vi "Get ni_measurements_v1_MeasurementParameters.vi"(8 "error in (no error)":errorcluster, 11 "gRPCid":T5) -> (0 "error out":errorcluster, 2 "package_templatemessage":T1, 3 "gRPCid out":T5)   [LabVIEW 2020, in "LoadRegulation.lvlib"]
uses:
  LoadRegulation.lvlib
  a51dd2a7-b5c1-4c09-9df4-8cd9d3bd0c19.vi
  ni_measurements_v1_ConfigurationParameter.ctl
  google_protobuf_Any.ctl
  ni_measurements_v1_Output.ctl
  ni_measurements_v1_MeasurementParameters.ctl
  <vilib>/gRPC/LabVIEW gRPC Library/Server API/typeDefs/grpcId.ctl
  <vilib>/gRPC/LabVIEW gRPC Library/gprc-lvsupport-release.lvlib
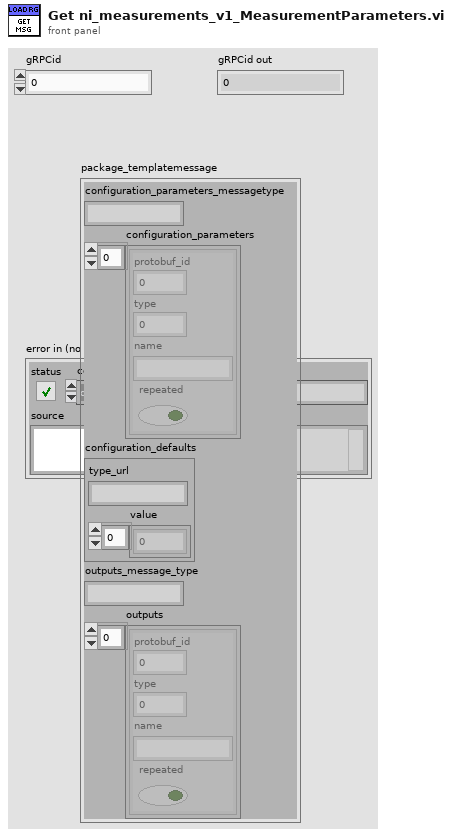
[diagram p1: front panel]
types:
  T1 = typedef "LoadRegulation.lvlib/ni_measurements_v1_MeasurementParameters.ctl" = cluster{"configuration_parameters_messagetype":string, "configuration_parameters":T2[], "configuration_defaults":T3, "outputs_message_type":string, "outputs":T4[]}
  T2 = typedef "LoadRegulation.lvlib/ni_measurements_v1_ConfigurationParameter.ctl" = cluster{"protobuf_id":u32, "type":i32, "name":string, "repeated":bool}
  T3 = typedef "LoadRegulation.lvlib/google_protobuf_Any.ctl" = cluster{"type_url":string, "value":u8[]}
  T4 = typedef "LoadRegulation.lvlib/ni_measurements_v1_Output.ctl" = cluster{"protobuf_id":u32, "type":i32, "name":string, "repeated":bool}
  T5 = typedef "gprc-lvsupport-release.lvlib/grpcId.ctl" = u64
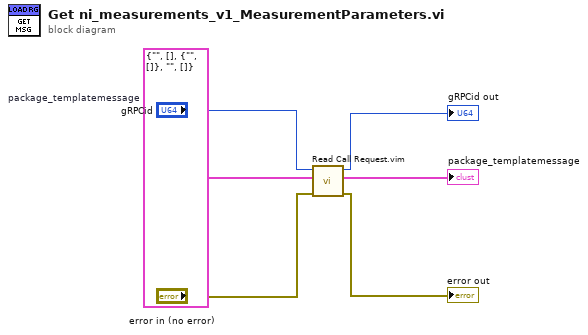
[diagram p0: block diagram]
diagram:
  w2 = T1 {"configuration_parameters_messagetype"="", "configuration_parameters"=[], "configuration_defaults"={"type_url"="", "value"=[]}, "outputs_message_type"="", "outputs"=[]}  # package_templatemessage
  n1 = call "Read Call Request.vim"("error in (no error)"="error in (no error)", "Data Type"=w2, "gRPCid in"="gRPCid") -> ("error out"=→"error out":errorcluster, "Request Data"=→"package_templatemessage":T1, "gRPCid out"=→"gRPCid out":T5)  [unwired: 6 in]
